vi "Converter to T&H.vi"(11 "buffer":u8[](array[numeric])) -> (2 "Numeric":dbl, 3 "Numeric 2":dbl)   [LabVIEW 2016]
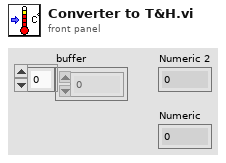
[diagram p1: front panel]
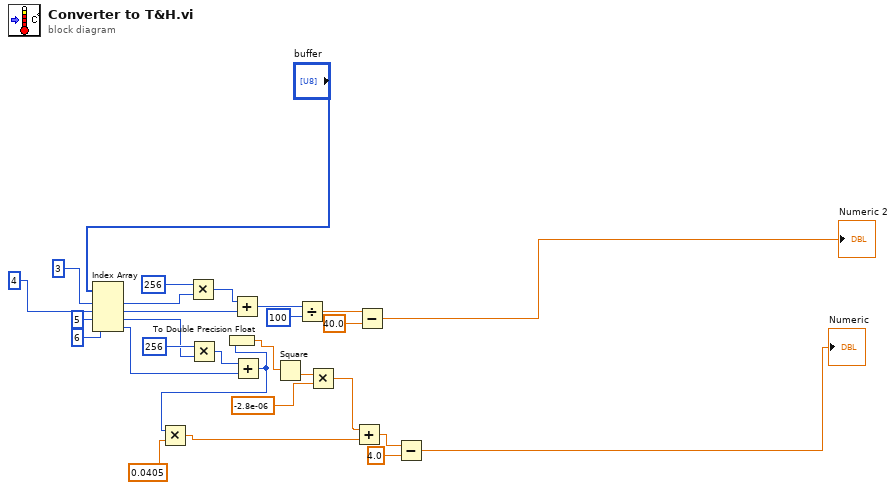
[diagram p0: block diagram]
diagram:
  n1 = Index Array(array="buffer", index #1=3 ("index"), index #2=4 ("index"), index #3=5 ("index"), index #4=6 ("index")) -> (element #1=w19:u8, element #2=w16:u8, element #3=w12:u8, element #4=w11:u8)
  n2 = Multiply(x=i16 256, y=w19) -> (x*y=w17:i16)
  n3 = Multiply(x=i16 256, y=w12) -> (x*y=w10:i16)
  n4 = Add(x=w17, y=w16) -> (x+y=w18:i16)
  n5 = Add(x=w10, y=w11) -> (x+y=w3:i16)
  n6 = Multiply(x=w3, y=0.0405) -> (x*y=w7:dbl)
  n7 = To Double Precision Float(number=w3) -> (double precision float=w2:dbl)
  n8 = Square(x=w2) -> (x^2=w4:dbl)
  n9 = Divide(x=w18, y=i16 100) -> (x/y=w22:dbl)
  n10 = Multiply(x=w4, y=-2.8e-06) -> (x*y=w1:dbl)
  n11 = Add(x=w1, y=w7) -> (x+y=w6:dbl)
  n12 = Subtract(x=w22, y=40.0) -> (x-y=→"Numeric 2":dbl)
  n13 = Subtract(x=w6, y=4.0) -> (x-y=→"Numeric":dbl)
